vi "ParsingTestStringData.vi"() -> ()   [LabVIEW 2020]
panel:
  in  "String":string="A+13.5424+24.5782+16.6670+15.4443+15.4443N2"
  out "Std. Mass Flow":string
  out "Array":string[](array[string])
  in  "stop":bool
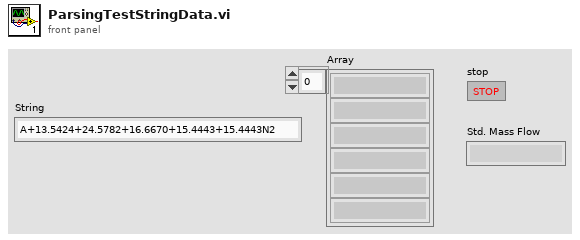
[diagram p1: front panel]
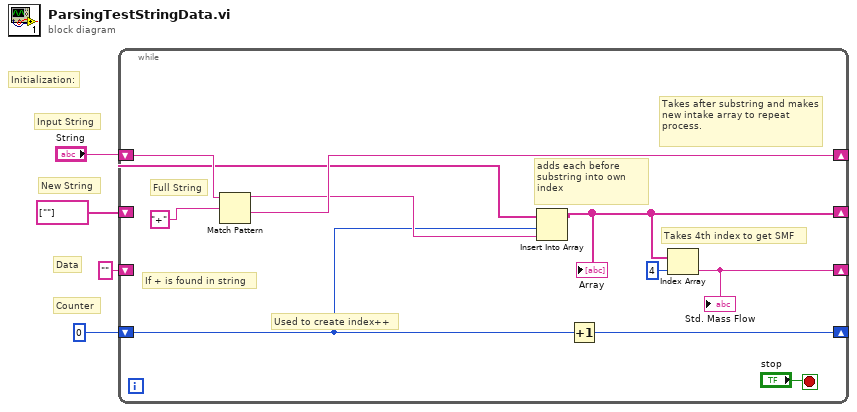
[diagram p0: block diagram]
diagram:
  # "Data"
  # "Initialization:"
  # "Counter"
  # "New String"
  # "Input String"
  n1 = while {
    shift-right: [w8] -> _
    shift-left: string[] [""] ("Array") -> [w11]
    shift-right: [w12] -> _
    shift-left: "String" -> [w13]
    shift-right: [w9] -> _
    shift-left: 0 -> [w5]
    shift-right: [w6] -> _
    shift-left: "" ("String") -> [_]
    stop <- "stop" stop-if-true
    # "Takes after substring and makes new intake array to repeat process."
    # "Used to create index++"
    # "Takes 4th index to get SMF"
    # "adds each before substring into own index"
    # "If + is found in string"
    # "Full String"
    n2 = Match Pattern(string=w13, regular expression="+") -> (before substring=w10:string, after substring=w12:string)  [unwired: 1 in, 2 out]
    n3 = Insert Into Array(array=w11, index=w5, new element=w10) -> (w8:string[])
    "Array" <- w8
    n4 = Increment(x=w5) -> (x+1=w9:i32)
    n5 = Index Array(array=w8, index=4) -> (element=w6:string)
    "Std. Mass Flow" <- w6
  }
